vi "CustomEvent.vi"() -> ()   [LabVIEW 2020]
panel:
  out "NewSN":i32
  in  "Product":cluster{"Name":string, "SN":i32}
  out "Name:":string
  in  "Format":bool
  in  "stop":bool
  # "Formated:"
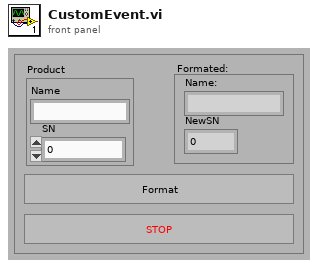
[diagram p1: front panel]
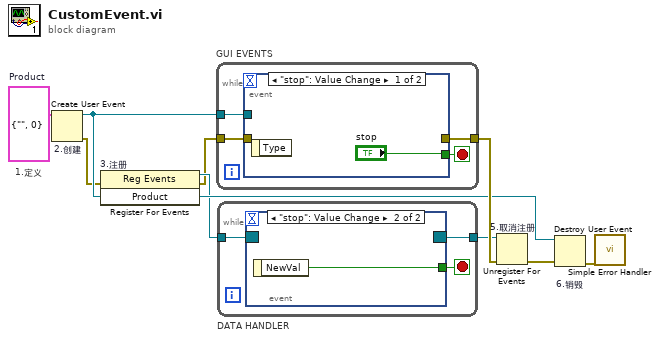
[diagram p0: block diagram]
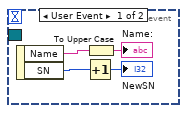
[diagram p2: hidden frame]
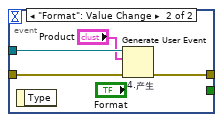
[diagram p3: hidden frame]
diagram:
  w6 = cluster{"Name":string, "SN":i32} {"Name"="", "SN"=0}  # Product
  # "1.定义"
  n1 = Create User Event "2.创建"(user event datatype=w6) -> (user event=w7:refnum<user-event>, error out=w2:errorcluster)  [unwired: 1 in]
  n2 = register-events "3.注册"(error in=w2, w7) -> (reference out=w3:refnum<event-registration>, error out=w1:errorcluster)  [unwired: 1 in]
  n3 = while "GUI EVENTS" {
    tunnel: w7 -> [w12]
    tunnel: [w11] -> w9
    tunnel: w1 -> [w10]
    stop <- w13 stop-if-true
    n4 = event shown="[0] \"stop\": Value Change" {
      selector: _ -> [_ _]
      dyn-events: _ -> [_ _]
      timeout: _ -> [_ _]
      tunnel: ["stop" _] -> w13
      tunnel: w12 -> [_ w18]
      tunnel: [_ w17] -> w11
      tunnel: w10 -> [_ w16]
      event "stop": Value Change {
        n5 = event-data() -> ()  [unwired: 1 in, 1 out]
      }
      event "Format": Value Change {
        n6 = event-data() -> ()  [unwired: 1 in, 1 out]
        n7 = Generate User Event "4.产生"(user event=w18, event data cluster="Product", error in=w16) -> (error out=w17:errorcluster)  [unwired: 1 in, 1 out]
      }
    }
  }
  n8 = while "DATA HANDLER" {
    tunnel: w3 -> [w21]
    tunnel: [w20] -> w4
    stop <- w19 stop-if-true
    n9 = event shown="[1] \"stop\": Value Change" {
      selector: w21 -> [_ _]
      dyn-events: [_ _] -> w20
      timeout: _ -> [_ _]
      tunnel: [_ w26] -> w19
      event User Event {
        n10 = event-data() -> ("Name"=w23:string, "SN"=w22:i32)  [unwired: 1 in]
        n11 = Increment(x=w22) -> (x+1=→"NewSN":i32)
        n12 = To Upper Case(1:w23) -> (0:→"Name:":string)
      }
      event "stop": Value Change {
        n13 = event-data() -> ("NewVal"=w26:bool)  [unwired: 1 in]
      }
    }
  }
  n14 = Unregister For Events "5.取消注册"(event registration refnum=w4, error in=w9) -> (error out=w8:errorcluster)
  n15 = Destroy User Event "6.销毁"(user event=w7, error in=w8) -> (error out=w5:errorcluster)
  n16 = call <vilib>:"Simple Error Handler.vi"("error in (no error)"=w5) -> ()  [unwired: 4 in, 5 out]
